vi "JSON Parse Errors.vi"(8 "error in (no error)":errorcluster, 11 "JSON command":string) -> (0 "error out":errorcluster, 2 "key found?":bool, 3 "error string (if existing)":string)   [LabVIEW 2023, in "horiba.lvlib" / "Communicator.lvclass"]
doc: "Parses the returned error into an LV error."
uses:
  Communicator.lvclass
  e4096ba3-d423-4a45-8b74-94d4f34800f8.vi
  <vilib>/JDP Science/JSONtext/Next JSON Value.vi
  <vilib>/JDP Science/JSONtext/String Subset.vi
  <vilib>/JDP Science/JSONtext/Parsing/Advance past next JSON Value (inlined COPY).vi
  <vilib>/JDP Science/JSONtext/Parsing/Advance past whitespace.vi
  <vilib>/JDP Science/JSONtext/Parsing/Advance past String.vi
  <vilib>/JDP Science/JSONtext/Parsing/Advance past Number.vi
  <vilib>/JDP Science/JSONtext/Parsing/Advance past Line Ending.vi
  <vilib>/JDP Science/JSONtext/Parsing/Parse Full Path or Item Name.vi
  <vilib>/JDP Science/JSONtext/Parsing/Advance past Array.vi
  <vilib>/JDP Science/JSONtext/Parsing/Advance past Object.vi
  <vilib>/JDP Science/JSONtext/support/Error Cluster From Code.vi
  <vilib>/JDP Science/JSONtext/Offset/Find Item Locations by Path.vi
  <vilib>/JDP Science/JSONtext/JSON text to Variant.vi
  <vilib>/JDP Science/JSONtext/LVClass Serializer/JSONtext LVClass Serializer.lvclass
  Communicator.lvclass/Communicator.ctl
  <vilib>/JDP Science/JSONtext/JSONtext.lvlib
panel:
  # "Connector Pane"
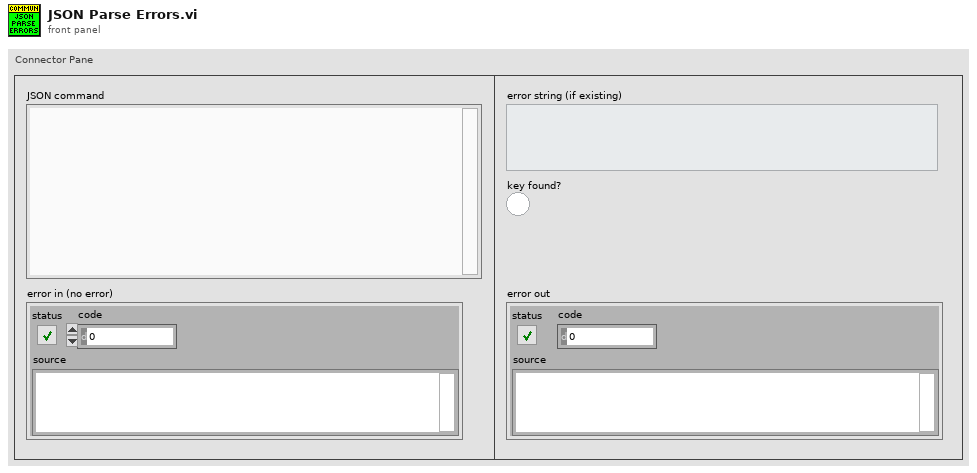
[diagram p1: front panel]
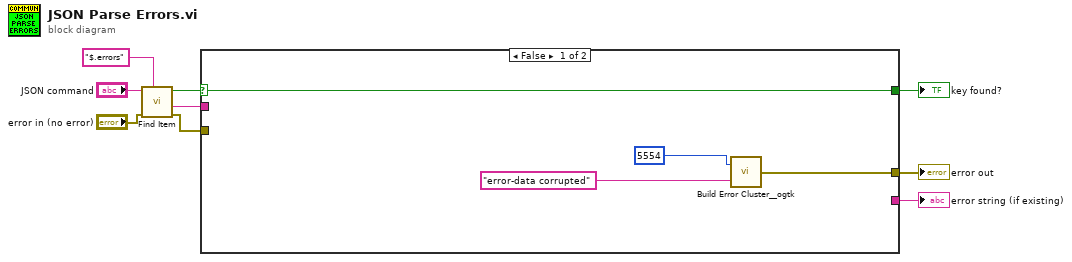
[diagram p0: block diagram]
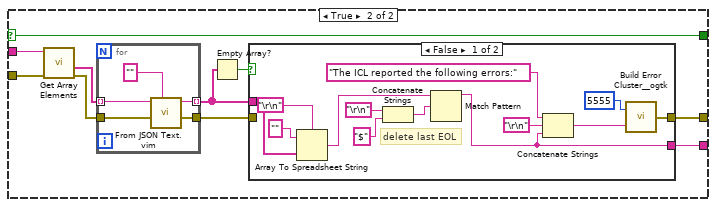
[diagram p2: hidden frame]
diagram:
  n1 = call <vilib>:"Find Item.vi"("$Path or Item Name"="$.errors", "error in (no error)"="error in (no error)", "JSON"="JSON command") -> ("error out"=w6:errorcluster, "<JSON>"=w7:string, "Found"=w5:bool)  [unwired: 5 in, 1 out]
  n2 = case shown="False" w5 {
    selector: w5 -> [w11 w16]
    tunnel: w7 -> [_ w23]
    tunnel: w6 -> [_ w22]
    tunnel: [w11 w16] -> w4
    tunnel: [w10 w15] -> w1
    tunnel: [_ w14] -> w3
    frame False {
      n3 = call <userlib>:"Build Error Cluster__ogtk.vi"("String to Prepend to source (\"\")"="error-data corrupted" ("String to Prepend to source (\"\")"), "code"=5554) -> ("error out"=w10:errorcluster)
    }
    frame True {
      n4 = call <vilib>:"Get Array Elements.vi"("error in (no error)"=w22, "JSON"=w23) -> ("error out"=w18:errorcluster, "<JSON>"=w21:string[])  [unwired: 7 in, 1 out]
      n5 = for {
        tunnel: w21 -> [w42] mode=indexing
        tunnel: [w40] -> w19 mode=indexing
        tunnel: w18 -> [w39]
        tunnel: [w38] -> w17
        n6 = call "From JSON Text.vim"("Data Type and Default Value"="", "error in (no error)"=w39, "JSON"=w42) -> ("error out"=w38:errorcluster, "Data out"=w40:string)  [unwired: 7 in]
      }
      n7 = Empty Array?(array=w19) -> (empty?=w20:bool)
      n8 = case shown="False" w20 {
        tunnel: w17 -> [_ w37]
        tunnel: [w32 w37] -> w15
        tunnel: w19 -> [w36 _]
        tunnel: [w27 _] -> w14
        frame False {
          # "delete last EOL"
          n9 = Array To Spreadsheet String(delimiter (Tab)="\r\n", array=w36, 3:"" ("format string")) -> (spreadsheet string=w28:string)
          n10 = Concatenate Strings("\r\n", "$" ("string")) -> (w24:string)
          n11 = Match Pattern(string=w28, regular expression=w24) -> (before substring=w27:string)  [unwired: 1 in, 3 out]
          n12 = Concatenate Strings("The ICL reported the following errors:" ("String to Prepend to source (\"\")"), "\r\n", w27) -> (w33:string)
          n13 = call <userlib>:"Build Error Cluster__ogtk.vi"("String to Prepend to source (\"\")"=w33, "code"=5555) -> ("error out"=w32:errorcluster)
        }
        frame True {
        }
      }
    }
  }
  "key found?" <- w4
  "error string (if existing)" <- w3
  "error out" <- w1
